vi "Buffer.Errors.vi"   [LabVIEW 2017, in "DSF Core.lvlib" / "Buffer.lvclass"]
uses:
  Buffer.lvclass
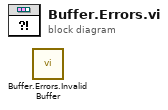
[diagram p0: block diagram]
diagram:
  n1 = call "Buffer.Errors.Invalid Buffer.vi"() -> ()  [unwired: 10 in, 2 out]
